vi "playSounds.vi"(1 "sounds":T1={"welcome sound"=path "C:/Users/wingX/Documents/WingXSVN/labview/daq test/sounds/welcome.wav", "play welcome"=TRUE, "got fly sound"=path "C:/Users/wingX/Documents/WingXSVN/labview/daq test/sounds/gotafly.wav", "play got fly"=FALSE, "discard sound"=path "C:/Users/wingX/Documents/WingXSVN/labview/daq test/sounds/blowingback.wav", "play discard"=FALSE, "finish sound"=path "C:/Users/wingX/Documents/WingXSVN/labview/daq test/sounds/finishedmeasuring.wav", "play finish"=TRUE, "inactivity alarm sound"=path "C:/Users/wingX/Documents/WingXSVN/labview/daq test/sounds/finishedmeasuring.wav", "play inactivity\nalarm"=TRUE}, 2 "task":T2(ring)=enum."blowing back") -> ()   [LabVIEW 2012]
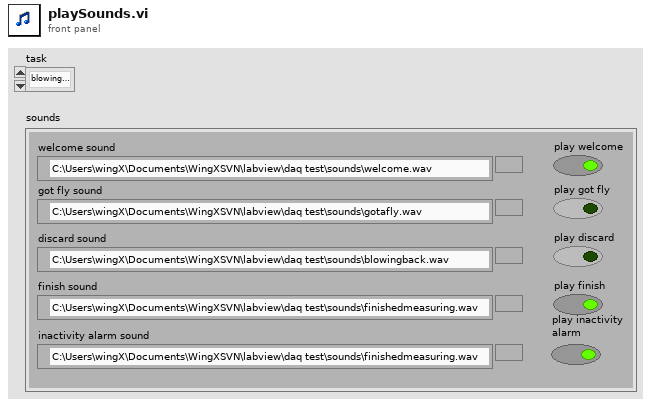
[diagram p1: front panel]
types:
  T1 = cluster{"welcome sound":path, "play welcome":bool, "got fly sound":path, "play got fly":bool, "discard sound":path, "play discard":bool, "finish sound":path, "play finish":bool, "inactivity alarm sound":path, "play inactivity\nalarm":bool}
  T2 = enum16{"waiting for fly", "closing gate", "fly in chamber", "taking decision", "keeping the fly", "blowing back", "activate flies"}
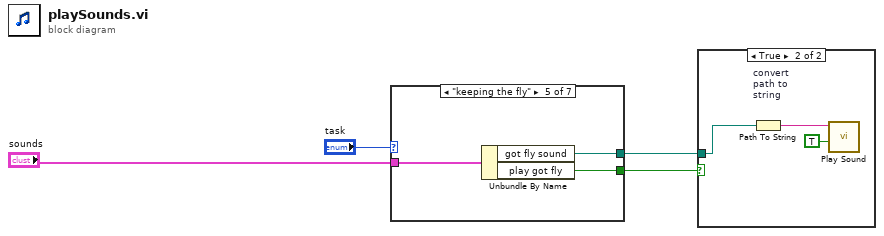
[diagram p0: block diagram]
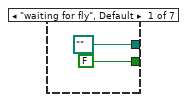
[diagram p2: hidden frame]
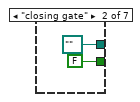
[diagram p3: hidden frame]
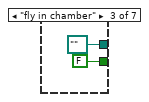
[diagram p4: hidden frame]
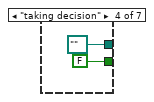
[diagram p5: hidden frame]
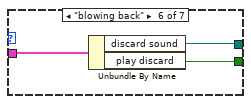
[diagram p6: hidden frame]
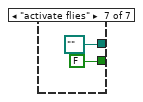
[diagram p7: hidden frame]
diagram:
  n1 = case shown="\"keeping the fly\"" "task" {
    tunnel: [path "" ("discard sound") path "" ("discard sound") path "" ("discard sound") path "" ("discard sound") w15 w18 path "" ("discard sound")] -> w3
    tunnel: [FALSE ("play discard") FALSE ("play discard") FALSE ("play discard") FALSE ("play discard") w14 w17 FALSE ("play discard")] -> w2
    tunnel: "sounds" -> [_ _ _ _ w13 w16 _]
    frame "waiting for fly", Default {
    }
    frame "closing gate" {
    }
    frame "fly in chamber" {
    }
    frame "taking decision" {
    }
    frame "keeping the fly" {
      n2 = Unbundle By Name(w13) -> ("got fly sound"=w15:path, "play got fly"=w14:bool)
    }
    frame "blowing back" {
      n3 = Unbundle By Name(w16) -> ("discard sound"=w18:path, "play discard"=w17:bool)
    }
    frame "activate flies" {
    }
  }
  n4 = case shown="True" w2 {
    tunnel: w3 -> [_ w22]
    frame False {
    }
    frame True {
      n5 = Path To String "convert\npath to\nstring"(path=w22) -> (string=w23:string)
      n6 = call "Play Sound.vi"("Asynchronous? (F)"=TRUE, "Sound Name"=w23) -> ()  [unwired: 3 in, 1 out]
    }
  }
